vi "To Default.vi"(8 "error in (no error)":errorcluster, 11 "Data in":refnum<class "Data.lvclass">) -> (0 "error dub":errorcluster, 3 "Data out":refnum<class "Data.lvclass">)   [LabVIEW 2020, in "Data.lvlib" / "Data.lvclass"]
doc: "Restore class data to the default value."
uses:
  Data.lvclass
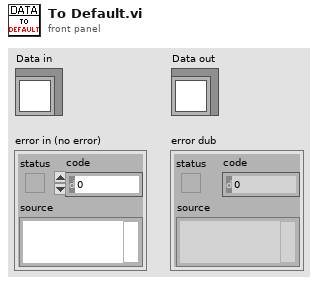
[diagram p1: front panel]
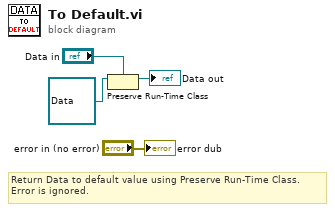
[diagram p0: block diagram]
diagram:
  # "Return Data to default value using Preserve Run-Time Class.\nError is ignored."
  n1 = Preserve Run-Time Class(object in=refnum<class "Data.lvclass"> refnum ("Data.lvlib:Data.lvclass"), 2:"Data in") -> (object out=→"Data out":refnum<class "Data.lvclass">)  [unwired: 1 in, 1 out]
  "error dub" <- "error in (no error)"
